vi "arm tune.vi"(0 "Tune Data":cluster{"Increment":bool, "Decrement":bool}, 3 "Setpoint":dbl, 4 "Save Tunes for Entire Match?":bool) -> (6 "Tuned Setpoint":dbl)   [LabVIEW 2013]
panel:
  # "Let drivers tune the setpoint of the arm to adapt for different ball sizes"
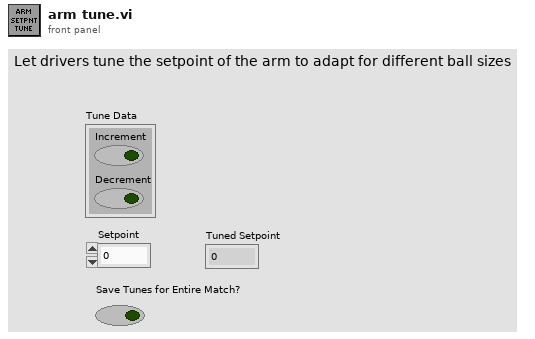
[diagram p1: front panel]
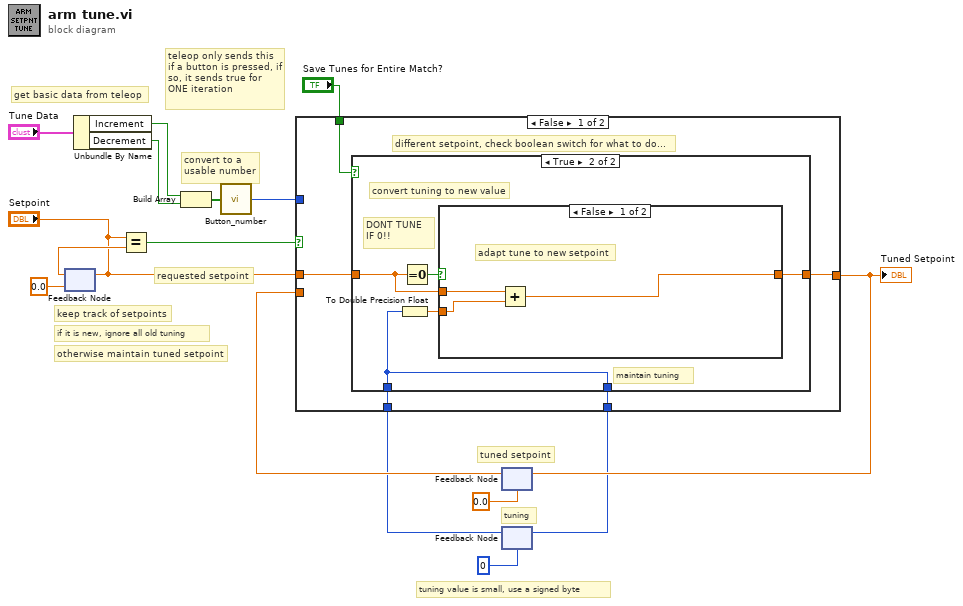
[diagram p0: block diagram]
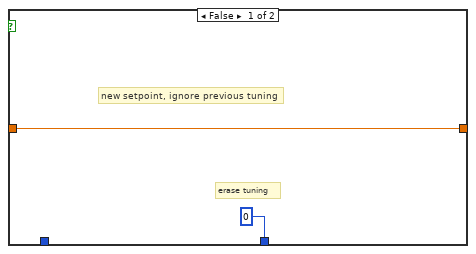
[diagram p2: hidden frame]
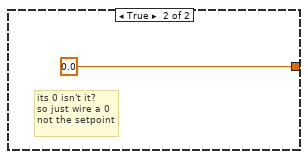
[diagram p3: hidden frame]
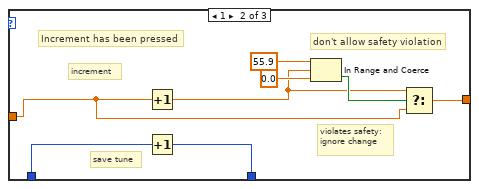
[diagram p5: hidden frame]
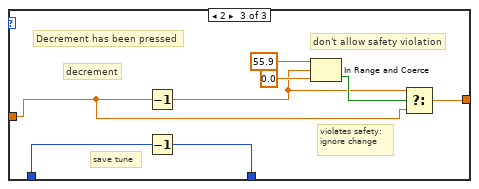
[diagram p6: hidden frame]
diagram:
  # "tuning value is small, use a signed byte"
  # "tuning"
  # "requested setpoint"
  # "tuned setpoint"
  # "otherwise maintain tuned setpoint"
  # "convert to a\nusable number"
  # "if it is new, ignore all old tuning"
  # "keep track of setpoints"
  # "teleop only sends this\nif a button is pressed, if\nso, it sends true for\nONE iteration"
  # "get basic data from teleop"
  n1 = feedback-in #1("Setpoint") -> ()
  n2 = feedback #1(0.0 ("Setpoint")) -> (w14:dbl)
  n3 = Unbundle By Name("Tune Data") -> ("Increment"=w13:bool, "Decrement"=w12:bool)
  n4 = Equal?(x="Setpoint", y=w14) -> (x = y?=w9:bool)
  n5 = Build Array(w13, w12) -> (w11:bool[])
  n6 = call "Button_number.vi"("Button Array"=w11) -> ("Button Pressed"=w10:i32)
  n7 = feedback #2(0.0) -> (w7:dbl)
  n8 = feedback #3(i8 0) -> (w2:i8)
  n9 = case shown="False" w9 {
    tunnel: w10 -> [_ w37]
    tunnel: "Setpoint" -> [w20 _]
    tunnel: w7 -> [_ w36]
    tunnel: [w19 w35] -> w6
    tunnel: "Save Tunes for Entire Match?" -> [w21 _]
    tunnel: w2 -> [w18 w34]
    tunnel: [w17 w33] -> w1
    frame False {
      # "different setpoint, check boolean switch for what to do..."
      n10 = case shown="True" w21 {
        tunnel: w20 -> [w23 w25]
        tunnel: [w23 w27] -> w19
        tunnel: w18 -> [_ w24]
        tunnel: [i8 0 w24] -> w17
        frame False {
          # "erase tuning"
          # "new setpoint, ignore previous tuning"
        }
        frame True {
          # "maintain tuning"
          # "DONT TUNE \nIF 0!!"
          # "convert tuning to new value"
          n11 = To Double Precision Float(number=w24) -> (double precision float=w26:dbl)
          n12 = Equal To 0?(x=w25) -> (x = 0?=w28:bool)
          n13 = case shown="False" w28 {
            tunnel: [w29 0.0] -> w27
            tunnel: w26 -> [w31 _]
            tunnel: w25 -> [w30 _]
            frame False {
              # "adapt tune to new setpoint"
              n14 = Add(x=w30, y=w31) -> (x+y=w29:dbl)
            }
            frame True {
              # "its 0 isn't it?\nso just wire a 0 \nnot the setpoint"
            }
          }
        }
      }
    }
    frame True {
      # "same setpoint, time to tune!"
      n15 = case shown="0, Default" w37 {
        tunnel: w36 -> [w39 w41 w49]
        tunnel: [w39 w40 w48] -> w35
        tunnel: w34 -> [w38 w47 w55]
        tunnel: [w38 w46 w54] -> w33
        frame 0, Default {
          # "leave tuning value alone"
          # "(aka last setpoint out)"
          # "nothing pressed, keep last TUNED value"
        }
        frame 1 {
          # "Increment has been pressed"
          # "violates safety:\nignore change"
          # "don't allow safety violation"
          # "save tune"
          # "increment"
          n16 = Increment(x=w41) -> (x+1=w42:dbl)
          n17 = Increment(x=w47) -> (x+1=w46:i8)
          n18 = In Range and Coerce(upper limit=55.9, x=w42, lower limit=0.0) -> (In Range?=w43:bool)  [unwired: 1 out]
          n19 = Select(t=w42, s=w43, f=w41) -> (s? t:f=w40:dbl)
        }
        frame 2 {
          # "Decrement has been pressed"
          # "decrement"
          # "save tune"
          # "violates safety:\nignore change"
          # "don't allow safety violation"
          n20 = Decrement(x=w49) -> (x-1=w50:dbl)
          n21 = Decrement(x=w55) -> (x-1=w54:i8)
          n22 = In Range and Coerce(upper limit=55.9, x=w50, lower limit=0.0) -> (In Range?=w51:bool)  [unwired: 1 out]
          n23 = Select(t=w50, s=w51, f=w49) -> (s? t:f=w48:dbl)
        }
      }
    }
  }
  "Tuned Setpoint" <- w6
  n24 = feedback-in #2(w6) -> ()
  n25 = feedback-in #3(w1) -> ()
